vi "1 port_Voltage Parameters.vi"(0 "Port Measurements":T3, 5 "Port Parametic Calculations":T2, 11 "Error In":errorcluster) -> (4 "Port Voltage Parametic Calculations":T1, 15 "Error Out":errorcluster)   [LabVIEW 2013]
uses:
  Controls/Port Measurements.ctl
  Controls/Port Capacitance Parametric Calculations.ctl
  Controls/Port Voltage Parametric Calculations.ctl
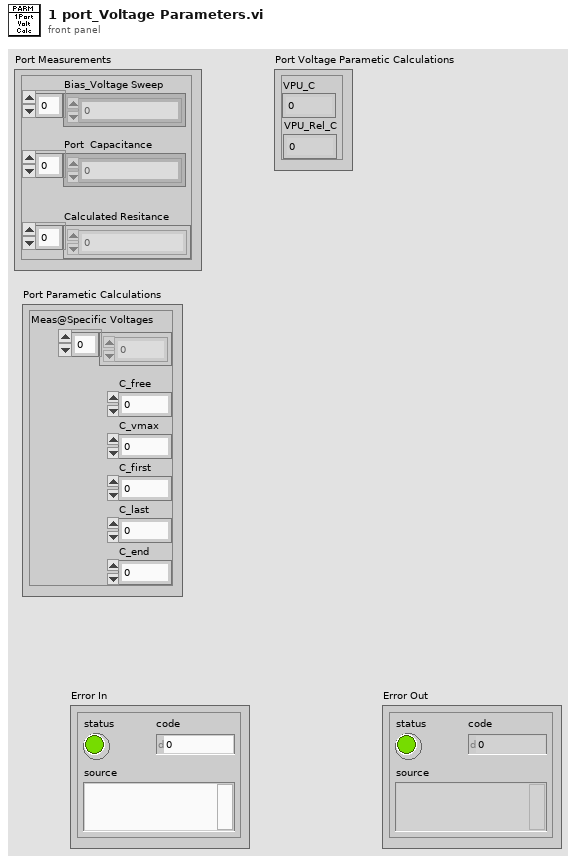
[diagram p1: front panel]
types:
  T1 = typedef "Port Voltage Parametric Calculations.ctl" = cluster{"VPU_C":dbl, "VPU_Rel_C":dbl}
  T2 = typedef "Port Capacitance Parametric Calculations.ctl" = cluster{"C_free":dbl, "C_vmax":dbl, "C_first":dbl, "C_last":dbl, "C_end":dbl, "Meas@Specific Voltages":dbl[]}
  T3 = typedef "Port Measurements.ctl" = cluster{"Bias_Voltage Sweep":dbl[], "Port  Capacitance":dbl[], "Calculated Resitance":dbl[]}
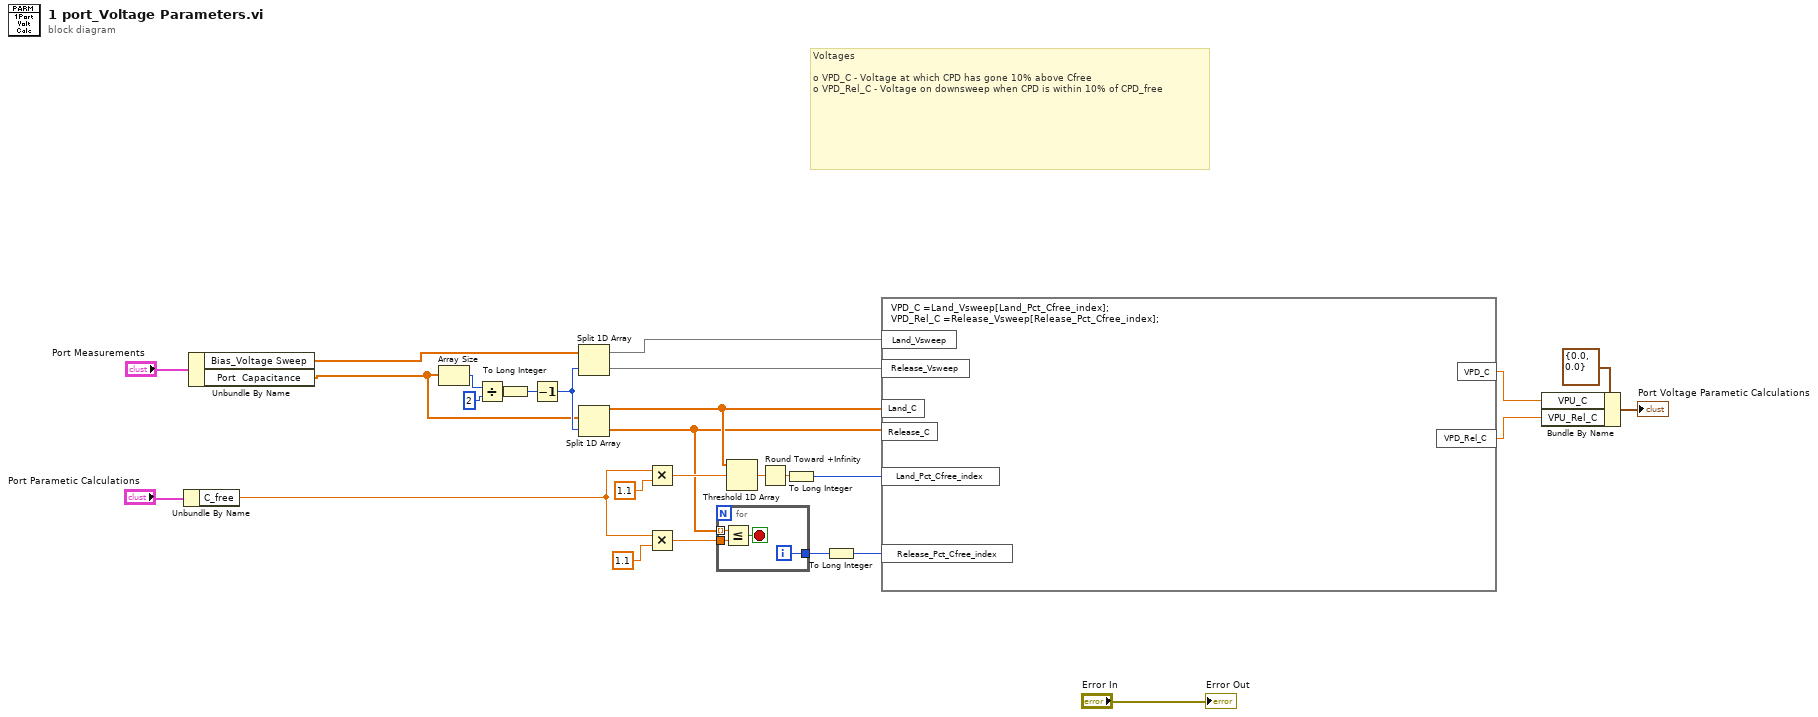
[diagram p0: block diagram]
diagram:
  # "Voltages\n\no\tVPD_C - Voltage at which CPD has gone 10% above Cfree\no\tVPD_Rel_C - Voltage on downsweep when CPD is within 10% of CPD_free"
  n1 = Unbundle By Name("Port Parametic Calculations") -> ("C_free"=w5:dbl)
  n2 = Unbundle By Name("Port Measurements") -> ("Bias_Voltage Sweep"=w8:dbl[], "Port  Capacitance"=w7:dbl[])
  n3 = Array Size(array=w7) -> (size(s)=w26:i32)
  n4 = Divide(x=w26, y=2) -> (x/y=w24:dbl)
  n5 = To Long Integer(number=w24) -> (32bit integer=w23:i32)
  n6 = Decrement(x=w23) -> (x-1=w16:i32)
  n7 = Split 1D Array(array=w8, index=w16) -> (first subarray=w15:dbl[], second subarray=w14:dbl[])
  n8 = Split 1D Array(array=w7, index=w16) -> (first subarray=w22:dbl[], second subarray=w12:dbl[])
  n9 = Multiply(x=w5, y=1.1) -> (x*y=w21:dbl)
  n10 = Multiply(x=w5, y=1.1) -> (x*y=w11:dbl)
  n11 = for {
    tunnel: [w32] -> w10
    tunnel: w12 -> [w31] mode=indexing
    tunnel: w11 -> [w30]
    i -> [w32]
    stop <- w29 stop-if-true
    n12 = Less Or Equal?(x=w31, y=w30) -> (x <= y?=w29:bool)
  }
  n13 = Threshold 1D Array(2:w21, 3:w22) -> (0:w28:dbl)  [unwired: 1 in]
  n14 = Round Toward +Infinity(x=w28) -> (ceil(x): smallest int >= x=w27:dbl)
  n15 = To Long Integer(number=w27) -> (32bit integer=w19:i32)
  n16 = To Long Integer(number=w10) -> (32bit integer=w18:i32)
  n17 = formula code="VPD_C =Land_Vsweep[Land_Pct_Cfree_index];\nVPD_Rel_C =Release_Vsweep[Release_Pct_Cfree_index];"("Land_C"=w22, "Release_C"=w12, "Land_Pct_Cfree_index"=w19, "Release_Pct_Cfree_index"=w18, "Land_Vsweep"=w15, "Release_Vsweep"=w14) -> ("VPD_C"=w3:dbl, "VPD_Rel_C"=w2:dbl)
  n18 = Bundle By Name(cluster=T1 {"VPU_C"=0.0, "VPU_Rel_C"=0.0} ("Port Voltage Parametic Calculations 2"), "VPU_C"=w3, "VPU_Rel_C"=w2) -> (→"Port Voltage Parametic Calculations":T1)
  "Error Out" <- "Error In"
